vi "Controller - State Process.vi"(8 "error in (no error)":errorcluster, 11 "View Model":T1) -> (0 "error out":errorcluster, 3 "View Model":T1)   [LabVIEW 2017]
doc: "Process current state of Car Wash controller"
uses:
  View Model/Controls/View Model.ctl
  Configuration Database/Controls/Config Model.ctl
  Configuration Database/Controls/Config Commands.ctl
  Configuration Database/Controls/Congif Data.ctl
  View Model/Controls/Shared Model.ctl
  Error Handler/Controls/Error Model.ctl
  Error Handler/Controls/Error Data.ctl
  Error Handler/Controls/Error Type.ctl
  Controls/Car Wash Model.ctl
  Controls/Controller Overhead.ctl
  Controls/Vehicle Location.ctl
  Controls/Car Wash States.ctl
  Controls/CarWash CMD.ctl
  Views/Wash Display Console View/Controls/Car Wash Indicators.ctl
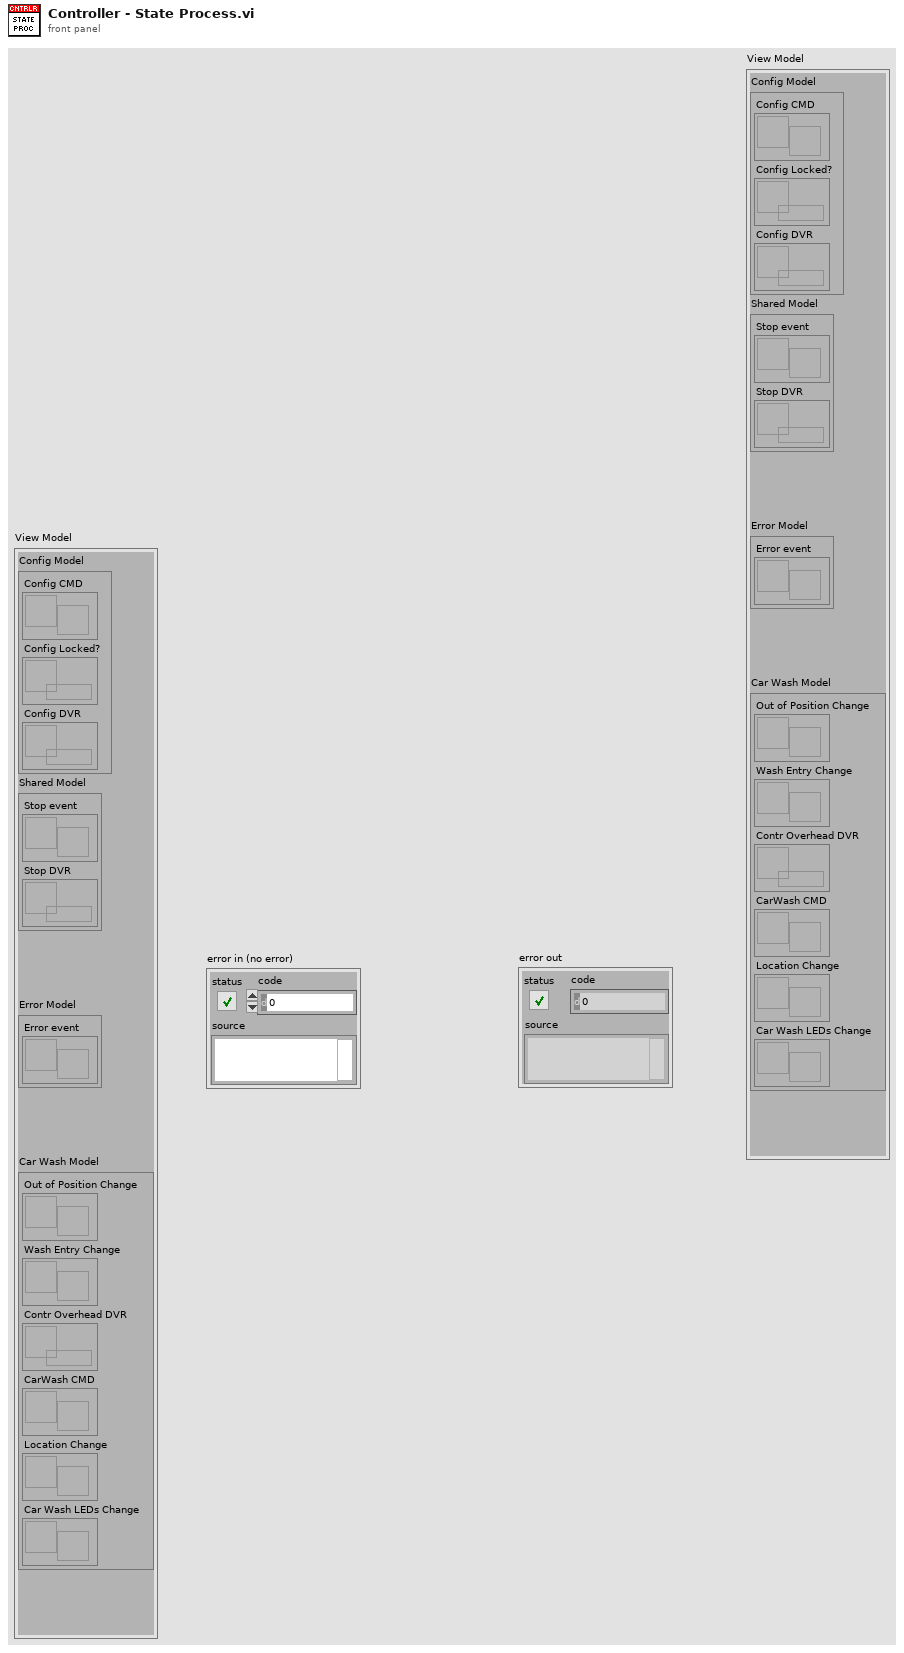
[diagram p1: front panel]
types:
  T1 = typedef "View Model.ctl" = cluster{"Config Model":T2, "Shared Model":T3, "Error Model":T4, "Car Wash Model":T5}
  T2 = typedef "Config Model.ctl" = cluster{"Config CMD":refnum<user-event>, "Config Locked?":refnum<data-value>, "Config DVR":refnum<data-value>}
  T3 = typedef "Shared Model.ctl" = cluster{"Stop event":refnum<user-event>, "Stop DVR":refnum<data-value>}
  T4 = typedef "Error Model.ctl" = cluster{"Error event":refnum<user-event>}
  T5 = typedef "Car Wash Model.ctl" = cluster{"Out of Position Change":refnum<user-event>, "Wash Entry Change":refnum<user-event>, "Contr Overhead DVR":refnum<data-value>, "CarWash CMD":refnum<user-event>, "Location Change":refnum<user-event>, "Car Wash LEDs Change":refnum<user-event>}
  T6 = typedef "Car Wash States.ctl" = enum16{"Initial", "Wait for start", "Start", "Wait for vehicle", "Wash Step Execution", "Wash Step/Cycle Complete", "Wash Exit", "Wash Abort/Terminate"}
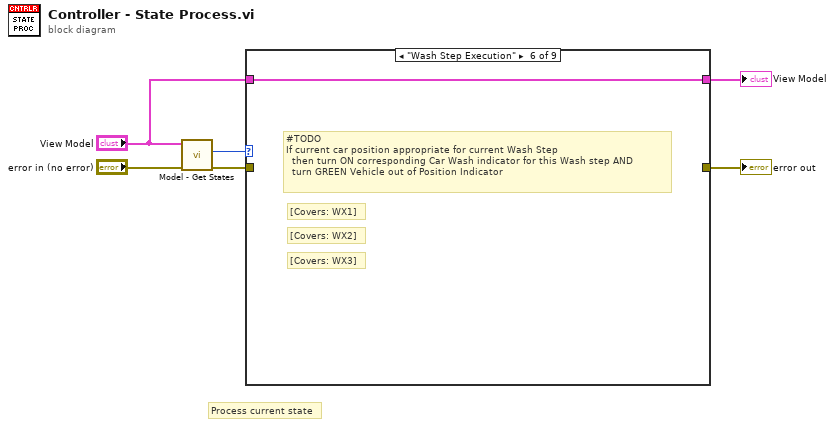
[diagram p0: block diagram]
diagram:
  # "Process current state"
  n1 = call "Model - Get States.vi"("error in (no error)"="error in (no error)", "View Model"="View Model") -> ("error out"=w3:errorcluster, "CarWash State"=w4:T6)  [unwired: 6 in, 2 out]
  n2 = case shown="\"Wash Step Execution\"" w4 {
    tunnel: "View Model" -> [w8 w9 w10 w11 w12 w13 w14 w15 w16]
    tunnel: [w8 w9 w10 w11 w12 w13 w14 w15 w16] -> w1
    tunnel: w3 -> [w7 _ _ _ _ _ _ _ _]
    tunnel: [w7 _ _ _ _ _ _ _ _] -> w2
    frame Default {
    }
    frame "Initial" {
    }
    frame "Wait for start" {
    }
    frame "Start" {
    }
    frame "Wait for vehicle" {
      # "[Covers: VS4]"
      # "#TODO\nWait untile user move the car to corresponding for active Wash step position.\nIf active step is last then wait for car moves to Exit"
      # "[Covers: VS3]"
      # "[Covers: VS2]"
      # "[Covers: VS1]"
      # "#TODO\n- Turn ON Car Wash indicator in accordance to active Wash Step\n- Turn RED Vehicle out of Position LED\n- Update Time Remaining indicator for the active Wash step's time"
    }
    frame "Wash Step Execution" {
      # "[Covers: WX3]"
      # "[Covers: WX2]"
      # "[Covers: WX1]"
      # "#TODO\nIf current car position appropriate for current Wash Step\n  then turn ON corresponding Car Wash indicator for this Wash step AND\n  turn GREEN Vehicle out of Position Indicator"
    }
    frame "Wash Step/Cycle Complete" {
    }
    frame "Wash Exit" {
    }
    frame "Wash Abort/Terminate" {
    }
  }
  "error out" <- w2
  "View Model" <- w1
